vi "LAC Cmd122_Output setting.vi"(6 "R/W (F:Read)":bool, 7 "timeout(ms)":u32=500, 8 "error in":errorcluster, 9 "Out port":enum16{"Serial", "Ethernet"}(ring), 10 "Out mode":enum16{"Stream", "I/O", "OFF"}(ring)=enum."I/O", 11 "VISA name in":refnum<visa-resource-name>) -> (0 "error out":errorcluster, 1 "readout":string, 3 "VISA name out":refnum<visa-resource-name>)   [LabVIEW 2014]
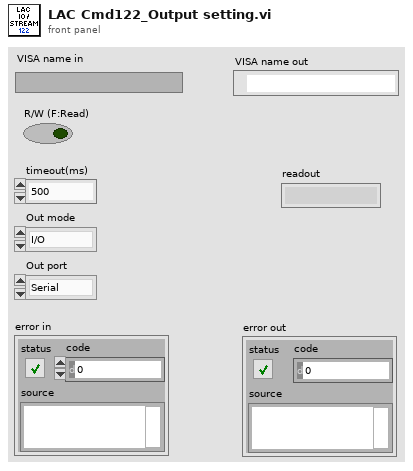
[diagram p1: front panel]
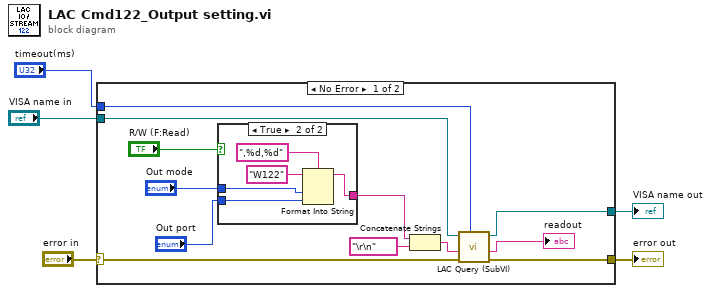
[diagram p0: block diagram]
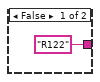
[diagram p2: hidden frame]
diagram:
  n1 = case shown="No Error" "error in" {
    selector: "error in" -> [w13 w25]
    tunnel: "VISA name in" -> [w15 w24]
    tunnel: [w17 w24] -> w4
    tunnel: [w16 w25] -> w3
    tunnel: "timeout(ms)" -> [w14 _]
    frame No Error {
      n2 = case shown="True" "R/W (F:Read)" {
        tunnel: ["R122" ("string") w22] -> w10
        tunnel: "Out port" -> [_ w21]
        tunnel: "Out mode" -> [_ w20]
        frame False {
        }
        frame True {
          n3 = Format Into String(format string=",%d,%d", initial string="W122" ("string"), w20, w21) -> (resulting string=w22:string)  [unwired: 1 in, 1 out]
        }
      }
      n4 = Concatenate Strings(w10, "\r\n" ("write buffer")) -> (w11:string)
      n5 = call "LAC Query (SubVI).vi"("timeout(ms)"=w14, "error in"=w13, "Command"=w11, "VISA name in"=w15) -> ("error out"=w16:errorcluster, "read buffer"=→"readout":string, "VISA name out"=w17:refnum<visa-resource-name>)  [unwired: 5 in]
    }
    frame Error {
    }
  }
  "VISA name out" <- w4
  "error out" <- w3
